vi "MakeExperimentFromTemplate.vi"(8 "error in (no error)":errorcluster, 10 "Target experiment directory":path, 11 "Source template directory":path) -> (0 "error out":errorcluster)   [LabVIEW 2017]
uses:
  <userlib>/_OpenG.lib/file/file.llb/File Exists - Scalar__ogtk.vi
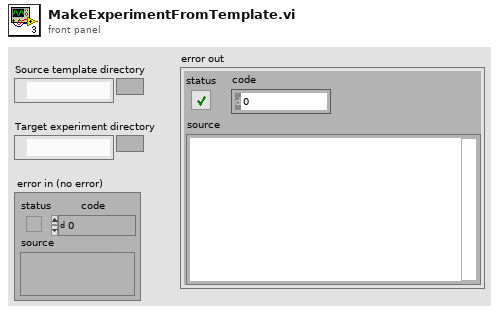
[diagram p1: front panel]
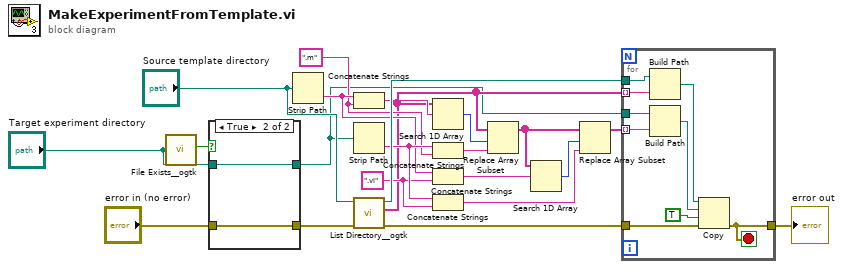
[diagram p0: block diagram]
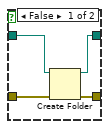
[diagram p2: hidden frame]
diagram:
  w15 = ".vi" ("string")
  w13 = ".m" ("string")
  n1 = call-poly <userlib>:"File Exists__ogtk.vi"("file path"="Target experiment directory") -> ("is directory"=w3:bool)  [unwired: 6 in, 1 out]
  n2 = case shown="True" w3 {
    tunnel: [w26 w28] -> w5
    tunnel: "Target experiment directory" -> [w25 w28]
    tunnel: "error in (no error)" -> [w24 w27]
    tunnel: [w23 w27] -> w1
    frame False {
      n3 = Create Folder(path (use dialog)=w25, error in=w24) -> (created path=w26:path, error out=w23:errorcluster)  [unwired: 1 in, 1 out]
    }
    frame True {
    }
  }
  n4 = Strip Path(path="Source template directory") -> (name=w14:string)  [unwired: 1 out]
  n5 = Concatenate Strings(w14, w13) -> (w20:string)
  n6 = Strip Path(path=w5) -> (name=w17:string)  [unwired: 1 out]
  n7 = call <userlib>:"List Directory__ogtk.vi"("error in (no error)"=w1, "directory path"="Source template directory") -> ("error out"=w10:errorcluster, "file names"=w8:string[], "dup directory path"=w22:path)  [unwired: 2 in, 1 out]
  n8 = Search 1D Array(1D array=w8, element=w20) -> (index of element=w19:i32)  [unwired: 1 in]
  n9 = Concatenate Strings(w17, w13) -> (w18:string)
  n10 = Concatenate Strings(w14, w15) -> (w7:string)
  n11 = Concatenate Strings(w17, w15) -> (w6:string)
  n12 = Replace Array Subset(array=w8, new element=w18, index=w19) -> (w12:string[])
  n13 = Search 1D Array(1D array=w12, element=w7) -> (index of element=w16:i32)  [unwired: 1 in]
  n14 = Replace Array Subset(array=w12, new element=w6, index=w16) -> (w11:string[])
  n15 = for {
    tunnel: w22 -> [w37]
    tunnel: w11 -> [w36] mode=indexing
    tunnel: w5 -> [w35]
    tunnel: w10 -> [w31]
    tunnel: [w30] -> w9
    tunnel: w8 -> [w29] mode=indexing
    stop <- w30 stop-if-true
    n16 = Build Path(base path=w37, name or relative path=w29) -> (appended path=w34:path)
    n17 = Build Path(base path=w35, name or relative path=w36) -> (appended path=w33:path)
    n18 = Copy(8:w31, 9:TRUE ("overwrite (F)"), 10:w33, 11:w34) -> (0:w30:errorcluster)  [unwired: 1 in, 2 out]
  }
  "error out" <- w9
